vi "main.vi"() -> ()   [LabVIEW 2012]
uses:
  number_of_sources.gbl
  shutter_timeout.gbl
  active_process.gbl
panel:
  in  "Clear elements":bool
  in  "Elements + Rates":cluster{"Elements":u16[], "Rates":sgl[]} {"Rates" min=0 step=0.1 format="%.1f"; "Elements" items=["none", "Ag", "AgBr", "AgCl", "Al", "Al2O3", "Al4C3", "AlF3", "AlN", "AlSb", "As", "As2Se3", "Au", "B", "B2O3", "B4C", "BN", "Ba", "BaF2", "BaN2O6", "BaO", "BaTiO3", "BaTiO3", "Be", "BeF2", "BeO", "Bi", "Bi2O3", "Bi2S3", "Bi2Se3", "Bi2Te3", "BiF3", "C", "C", "C8H8", "Ca", "CaF2", "CaO", "CaO-SiO2", "CaSO4", "CaTiO3", "CaWO4", "Cd", "CdF2", "CdO", "CdS", "CdSe", "CdTe", "Ce", "CeF3", "CeO2", "Co", "CoO", "Cr", "Cr2O3", "Cr3C2", "CrB", "Cs", "Cs2SO4", "CsBr", "CsCl", "CsI", "Cu", "Cu2O", "Cu2S", "Cu2S", "CuS", "Dy", "DY2O3", "Er", "Er2O3", "Eu", "EuF2", "Fe", "Fe2O3", "FeO", "FeS", "Ga", "Ga2O3", "GaAs", "GaN", "GaP", "GaSb", "Gd", "Gd2O3", "Ge", "Ge3N2", "GeO2", "GeTe", "Hf", "HfB2", "HfC", "HfN", "HfO2", "HfSi2", "Hg", "Ho", "Ho2O3", "In", "In2O3", "In2Se3", "In2Te3", "InAs", "InP", "InSb", "Ir", "K", "KBr", "KCl", "KF", "KI", "La", "La2O3", "LaB6", "LaF3", "Li", "LiBr", "LiF", "LiNbO3", "Lu", "Mg", "MgAl2O4", "MgAl2O6", "MgF2", "MgO", "Mn", "MnO", "MnS", "Mo", "Mo2C", "MoB2", "MoO3", "MoS2", "Na", "Na3AlF6", "Na5Al3F14", "NaBr", "NaCl", "NaClO3", "NaF", "NaNO3", "Nb", "Nb2O3", "Nb2O5", "NbB2", "NbC", "NbN", "Nd", "Nd2O3", "NdF3", "Ni", "NiCr", "NiCrFe", "NiFe", "NiFeMo", "NiO", "P3N5", "Pb", "PbCl2", "PbF2", "PbO", "PbS", "PbSe", "PbSnO3", "PbTe", "Pd", "PdO", "Po", "Pr", "Pr2O3", "Pt", "PtO2", "Ra", "Rb", "RbI", "Re", "Rh", "Ru", "S8", "Sb", "Sb2O3", "Sb2S3", "Sc", "Sc2O3", "Se", "Si", "Si3N4", "SiC", "SiO", "SiO2", "Sm", "Sm2O3", "Sn", "SnO2", "SnS", "SnSe", "SnTe", "Sr", "SrF2", "SrO", "Ta", "Ta2O5", "TaB2", "TaC", "TaN", "Tb", "Tc", "Te", "TeO2", "Th", "ThF4", "ThO2", "ThOF2", "Ti", "Ti2O3", "TiB2", "TiC", "TiN", "TiO", "TiO2", "Tl", "TlBr", "TlCl", "TlI", "U", "U3O8", "U4O9", "UO2", "V", "V2O5", "VB2", "VC", "VN", "VO2", "W", "WB2", "WC", "WO3", "WS2", "WSi2", "Y", "Y2O3", "Yb", "Yb2O3", "Zn", "Zn3Sb2", "ZnF2", "ZnO", "ZnS", "ZnSe", "ZnTe", "Zr", "ZrB2", "ZrC", "ZrN", "ZrO2"]}
  in  "Update":bool
  in  "Quit":bool
  in  "Main Menu":cluster{"Deposition":bool, "Deposition 2":bool}
  # "version 1.0.2"
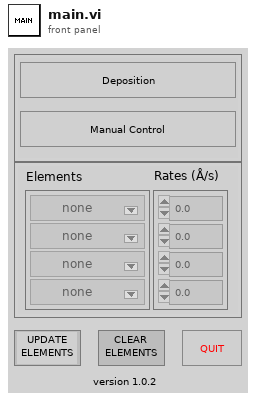
[diagram p1: front panel]
types:
  T1 = cluster{"Active process":i32, "Shutter timeout (ms)":u32, "Number of sources":i32}
  T2 = cluster{"Elements":u16[][], "TD":bool[], "Value":sgl[], "Repeats":i32}[]
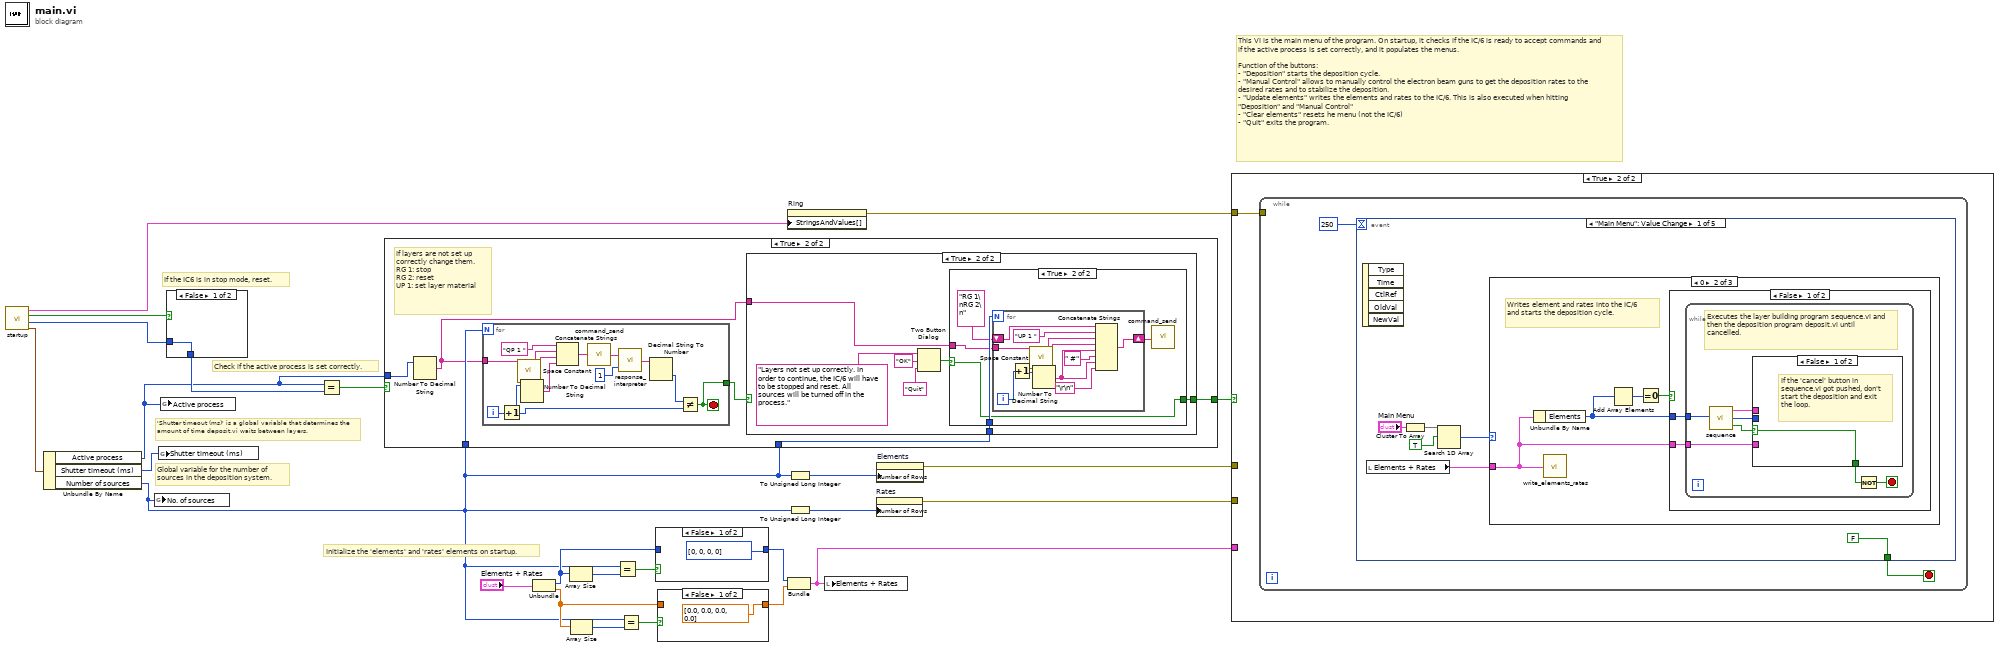
[diagram p0: block diagram]
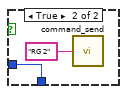
[diagram p2: hidden frame]
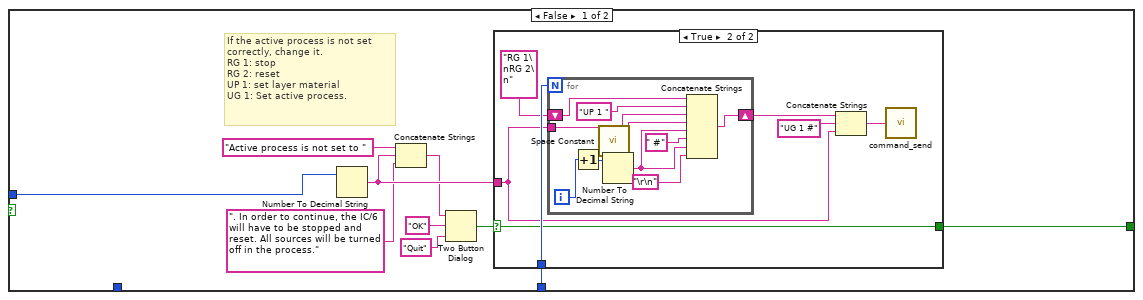
[diagram p3: hidden frame]
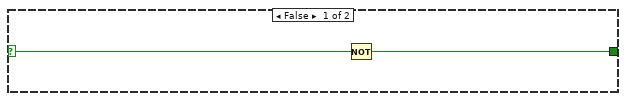
[diagram p5: hidden frame]
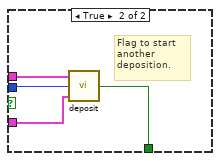
[diagram p9: hidden frame]
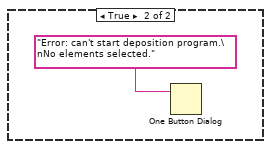
[diagram p10: hidden frame]
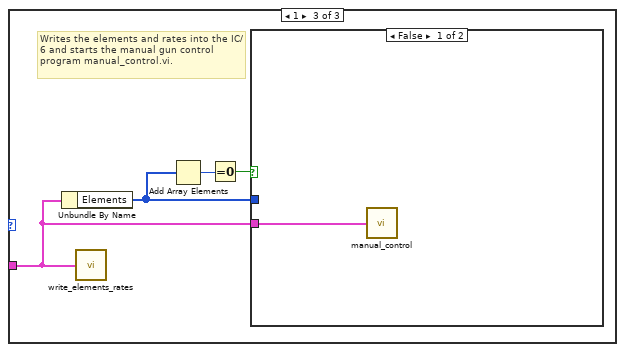
[diagram p11: hidden frame]
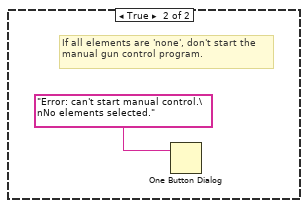
[diagram p12: hidden frame]
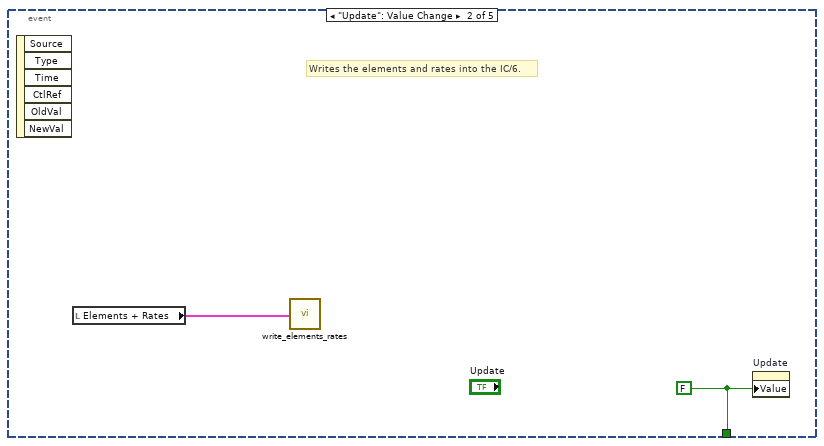
[diagram p13: hidden frame]
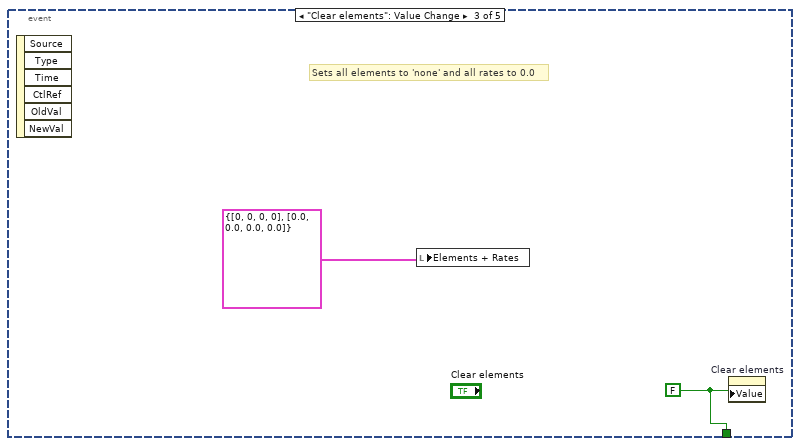
[diagram p14: hidden frame]
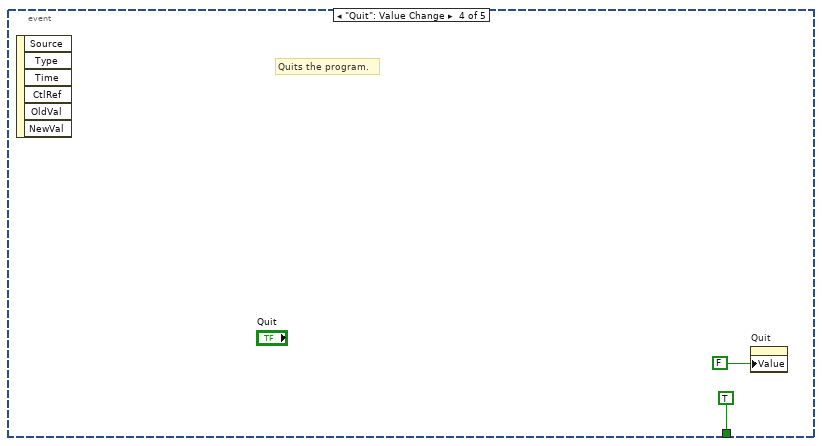
[diagram p15: hidden frame]
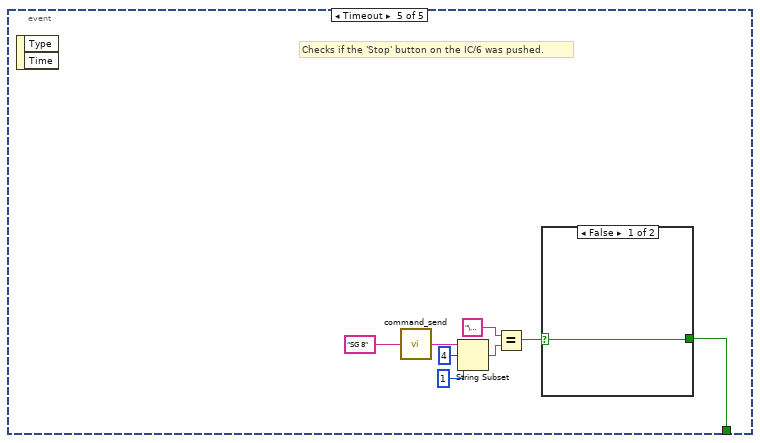
[diagram p16: hidden frame]
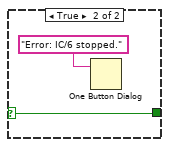
[diagram p17: hidden frame]
diagram:
  # "'Shutter timeout (ms)' is a global variable that determines the amount of time deposit.vi waits between layers."
  # "Global variable for the number of sources in the deposition system."
  # "This VI is the main menu of the program. On startup, it checks if the IC/6 is ready to accept commands and if the active process is set correctly, and it populates the menus.\n\nFunction of the buttons:\n- \"Deposition\" starts the deposition cycle.\n- \"Manual Control\" allows to manually control the electron beam guns to get the deposition rates to the desired rates and to stabilize the deposition.\n- \"Update elements\" writes the elements and rates to the IC/6. This is also executed when hitting \"Deposition\" and \"Manual Control\"\n- \"Clear elements\" resets he menu (not the IC/6)\n- \"Quit\" exits the program."
  # "Check if the active process is set correctly."
  # "If the IC6 is in stop mode, reset."
  # "Initialize the 'elements' and 'rates' elements on startup."
  n1 = call "startup.vi"() -> ("System parameters"=w9:T1, "Active process at IC6"=w10:i32, "Stop?"=w11:bool, "Elements+Rates ring items"=w12:cluster{"Element":string, "Value":u16}[])
  n2 = Unbundle By Name(w9) -> ("Active process"=w5:i32, "Shutter timeout (ms)"=w8:u32, "Number of sources"=w1:i32)
  n3 = global write "number_of_sources.gbl" "No. of sources"(w1) -> ()
  n4 = global write "shutter_timeout.gbl" "Shutter timeout (ms)"(w8) -> ()
  n5 = global write "active_process.gbl" "Active process"(w5) -> ()
  n6 = case shown="False" w11 {
    tunnel: w10 -> [w26 w27]
    tunnel: [w26 w27] -> w7
    frame False {
    }
    frame True {
      n7 = call "command_send.vi"("Commands"="RG 2") -> ()  [unwired: 1 out]
    }
  }
  n8 = Equal?(x=w5, y=w7) -> (x = y?=w20:bool)
  n9 = case shown="True" w20 {
    tunnel: [w35 w61] -> w17
    tunnel: w5 -> [w32 w62]
    tunnel: w1 -> [w29 w60]
    tunnel: w1 -> [_ w58]
    frame False {
      # "If the active process is not set\ncorrectly, change it.\nRG 1: stop\nRG 2: reset\nUP 1: set layer material\nUG 1: Set active process."
      n10 = Number To Decimal String(number=w32) -> (decimal integer string=w33:string)  [unwired: 1 in]
      n11 = Concatenate Strings("Active process is not set to ", w33, ". In order to continue, the IC/6 will have to be stopped and reset. All sources will be turned off in the process.") -> (w30:string)
      n12 = Two Button Dialog(message=w30, 1:"Quit", 2:"OK") -> (T button?=w36:bool)
      n13 = case shown="True" w36 {
        selector: w36 -> [w39 w45]
        tunnel: [w39 w45] -> w35
        tunnel: w33 -> [_ w40]
        tunnel: w29 -> [_ w46]
        frame False {
        }
        frame True {
          n14 = for {
            N: w46 -> [_]
            shift-right: [w56] -> w43
            shift-left: "RG 1\nRG 2\n" -> [w50]
            tunnel: w40 -> [w48]
            i -> [w54]
            n15 = Increment(x=w54) -> (x+1=w55:i32)
            n16 = call <vilib>:"Space Constant.vi"() -> ("String"=w47:string)
            n17 = Number To Decimal String(number=w55) -> (decimal integer string=w52:string)  [unwired: 1 in]
            n18 = Concatenate Strings(w50, "UP 1 ", w48, w47, w52, " #", w52, "\r\n") -> (w56:string)
          }
          n19 = Concatenate Strings(w43, "UG 1 #", w40) -> (w42:string)
          n20 = call "command_send.vi"("Commands"=w42) -> ()  [unwired: 1 out]
        }
      }
    }
    frame True {
      # "If layers are not set up correctly change them.\nRG 1: stop\nRG 2: reset\nUP 1: set layer material"
      n21 = Number To Decimal String(number=w62) -> (decimal integer string=w57:string)  [unwired: 1 in]
      n22 = for {
        N: w58 -> [_]
        tunnel: w57 -> [w70]
        tunnel: [w63] -> w59
        i -> [w74]
        stop <- w63 stop-if-true
        n23 = Increment(x=w74) -> (x+1=w64:i32)
        n24 = call <vilib>:"Space Constant.vi"() -> ("String"=w72:string)
        n25 = Number To Decimal String(number=w64) -> (decimal integer string=w73:string)  [unwired: 1 in]
        n26 = Concatenate Strings("QP 1 ", w70, w72, w73) -> (w67:string)
        n27 = call "command_send.vi"("Commands"=w67) -> ("Response"=w68:string)
        n28 = call "response_interpreter.vi"("Response type"=u16 1, "Response hex"=w68) -> ("Response (readable)"=w66:string)
        n29 = Decimal String To Number(string=w66) -> (number=w65:i32)  [unwired: 2 in, 1 out]
        n30 = Not Equal?(x=w65, y=w64) -> (x != y?=w63:bool)
      }
      n31 = case shown="True" w59 {
        selector: w59 -> [w76 _]
        tunnel: w60 -> [_ w83]
        tunnel: [w75 w82] -> w61
        tunnel: w57 -> [_ w77]
        frame False {
          n32 = Not(x=w76) -> (.not. x?=w75:bool)
        }
        frame True {
          n33 = Two Button Dialog(message="Layers not set up correctly. In order to continue, the IC/6 will have to be stopped and reset. All sources will be turned off in the process.", 1:"Quit", 2:"OK") -> (T button?=w79:bool)
          n34 = case shown="True" w79 {
            selector: w79 -> [w84 w86]
            tunnel: w83 -> [_ w88]
            tunnel: [w84 w86] -> w82
            tunnel: w77 -> [_ w85]
            frame False {
            }
            frame True {
              n35 = for {
                N: w88 -> [_]
                shift-right: [w99] -> w89
                shift-left: "RG 1\nRG 2\n" -> [w93]
                tunnel: w85 -> [w91]
                i -> [w97]
                n36 = Increment(x=w97) -> (x+1=w98:i32)
                n37 = call <vilib>:"Space Constant.vi"() -> ("String"=w90:string)
                n38 = Number To Decimal String(number=w98) -> (decimal integer string=w95:string)  [unwired: 1 in]
                n39 = Concatenate Strings(w93, "UP 1 ", w91, w90, w95, " #", w95, "\r\n") -> (w99:string)
              }
              n40 = call "command_send.vi"("Commands"=w89) -> ()  [unwired: 1 out]
            }
          }
        }
      }
    }
  }
  n41 = Unbundle("Elements + Rates") -> ("Elements"=w3:u16[], "Rates"=w2:sgl[])
  n42 = Array Size(array=w3) -> (size(s)=w18:i32)
  n43 = Array Size(array=w2) -> (size(s)=w19:i32)
  n44 = Equal?(x=w1, y=w18) -> (x = y?=w23:bool)
  n45 = Equal?(x=w1, y=w19) -> (x = y?=w24:bool)
  n46 = case shown="False" w23 {
    tunnel: w3 -> [_ w101]
    tunnel: [u16[] [0, 0, 0, 0] w101] -> w21
    frame False {
    }
    frame True {
    }
  }
  n47 = case shown="False" w24 {
    tunnel: w2 -> [_ w103]
    tunnel: [sgl[] [0.0, 0.0, 0.0, 0.0] w103] -> w22
    frame False {
    }
    frame True {
    }
  }
  n48 = property on="Ring" class="Ring (strict)"("StringsAndValues[]"=w12) -> (error out=w16:errorcluster)  [unwired: 2 in, 1 out]
  n49 = Bundle("Elements"=w21, "Rates"=w22) -> (w13:cluster{"Elements":u16[], "Rates":sgl[]})  [unwired: 1 in]
  n50 = To Unsigned Long Integer(number=w1) -> (unsigned 32bit integer=w4:u32)
  n51 = To Unsigned Long Integer(number=w1) -> (unsigned 32bit integer=w6:u32)
  n52 = local write "Elements + Rates"(w13) -> ()
  n53 = property on="Rates" class="Arr (strict)"("Number of Rows"=w6) -> (error out=w14:errorcluster)  [unwired: 2 in, 1 out]
  n54 = property on="Elements" class="Arr (strict)"("Number of Rows"=w4) -> (error out=w15:errorcluster)  [unwired: 2 in, 1 out]
  n55 = case shown="True" w17 {
    tunnel: w16 -> [_ w104]
    tunnel: w15 -> [_ _]
    tunnel: w14 -> [_ _]
    tunnel: w13 -> [_ _]
    frame False {
    }
    frame True {
      n56 = while {
        tunnel: w104 -> [_]
        stop <- w106 stop-if-true
        n57 = event shown="[0] \"Main Menu\": Value Change" {
          selector: _ -> [_ _ _ _ _]
          dyn-events: _ -> [_ _ _ _ _]
          timeout: 250 -> [_ _ _ _ _]
          tunnel: [FALSE w138 w140 TRUE w145] -> w106
          event "Main Menu": Value Change {
            n58 = event-data() -> ()  [unwired: 1 in, 5 out]
            n59 = local read "Elements + Rates"() -> (w107:cluster{"Elements":u16[], "Rates":sgl[]})
            n60 = Cluster To Array(cluster="Main Menu") -> (array=w111:bool[])
            n61 = Search 1D Array(1D array=w111, element=TRUE) -> (index of element=w109:i32)  [unwired: 1 in]
            n62 = case shown="0" w109 {
              tunnel: w107 -> [_ w113 w132]
              frame -1, Default {
              }
              frame 0 {
                # "Writes element and rates into the IC/6 and starts the deposition cycle."
                n63 = Unbundle By Name(w113) -> ("Elements"=w114:u16[])
                n64 = call "write_elements_rates.vi"("Elements + Rates"=w113) -> ()
                n65 = Add Array Elements(numeric array=w114) -> (sum=w115:u16)
                n66 = Equal To 0?(x=w115) -> (x = 0?=w116:bool)
                n67 = case shown="False" w116 {
                  tunnel: w114 -> [w118 _]
                  tunnel: w113 -> [w117 _]
                  frame False {
                    n68 = while {
                      tunnel: w118 -> [w120]
                      tunnel: w117 -> [w119]
                      stop <- w124 stop-if-true
                      # "Executes the layer building program sequence.vi and then the deposition program deposit.vi until cancelled."
                      n69 = call "sequence.vi"("Elements@IC6"=w120) -> ("Output Array"=w123:T2, "# of layers"=w121:i32, "Start/Cancel"=w122:bool)
                      n70 = case shown="False" w122 {
                        selector: w122 -> [w126 _]
                        tunnel: [w126 w129] -> w125
                        tunnel: w123 -> [_ w130]
                        tunnel: w121 -> [_ w128]
                        tunnel: w119 -> [_ w127]
                        frame False {
                          # "If the 'cancel' button in sequence.vi got pushed, don't start the deposition and exit the loop."
                        }
                        frame True {
                          # "Flag to start another deposition."
                          n71 = call "deposit.vi"("Elements+Rates"=w127, "# of units"=w128, "Input array"=w130) -> ("Deposit again?"=w129:bool)
                        }
                      }
                      n72 = Not(x=w125) -> (.not. x?=w124:bool)
                    }
                  }
                  frame True {
                    n73 = One Button Dialog(message="Error: can't start deposition program.\nNo elements selected.") -> ()  [unwired: 1 in, 1 out]
                  }
                }
              }
              frame 1 {
                # "Writes the elements and rates into the IC/6 and starts the manual gun control program manual_control.vi."
                n74 = Unbundle By Name(w132) -> ("Elements"=w133:u16[])
                n75 = call "write_elements_rates.vi"("Elements + Rates"=w132) -> ()
                n76 = Add Array Elements(numeric array=w133) -> (sum=w135:u16)
                n77 = Equal To 0?(x=w135) -> (x = 0?=w134:bool)
                n78 = case shown="False" w134 {
                  tunnel: w133 -> [_ _]
                  tunnel: w132 -> [w136 _]
                  frame False {
                    n79 = call "manual_control.vi"("Elements+Rates"=w136) -> ()
                  }
                  frame True {
                    # "If all elements are 'none', don't start the manual gun control program."
                    n80 = One Button Dialog(message="Error: can't start manual control.\nNo elements selected.") -> ()  [unwired: 1 in, 1 out]
                  }
                }
              }
            }
          }
          event "Update": Value Change {
            w138 = FALSE
            # "Writes the elements and rates into the IC/6."
            n81 = event-data() -> ()  [unwired: 1 in, 6 out]
            n82 = local read "Elements + Rates"() -> (w139:cluster{"Elements":u16[], "Rates":sgl[]})
            n83 = call "write_elements_rates.vi"("Elements + Rates"=w139) -> ()
            n84 = property on="Update" class="Bool (strict)"("Value"=w138) -> ()  [unwired: 2 in, 2 out]
          }
          event "Clear elements": Value Change {
            w140 = FALSE
            # "Sets all elements to 'none' and all rates to 0.0"
            n85 = event-data() -> ()  [unwired: 1 in, 6 out]
            n86 = local write "Elements + Rates"(cluster{u16[], sgl[]} {[0, 0, 0, 0], [0.0, 0.0, 0.0, 0.0]}) -> ()
            n87 = property on="Clear elements" class="Bool (strict)"("Value"=w140) -> ()  [unwired: 2 in, 2 out]
          }
          event "Quit": Value Change {
            # "Quits the program."
            n88 = event-data() -> ()  [unwired: 1 in, 6 out]
            n89 = property on="Quit" class="Bool (strict)"("Value"=FALSE) -> ()  [unwired: 2 in, 2 out]
          }
          event Timeout {
            # "Checks if the 'Stop' button on the IC/6 was pushed."
            n90 = event-data() -> ()  [unwired: 1 in, 2 out]
            n91 = call "command_send.vi"("Commands"="SG 8") -> ("Response"=w150:string)
            n92 = String Subset(string=w150, offset (0)=4, length (rest)=1) -> (substring=w147:string)
            n93 = Equal?(x="\u0006", y=w147) -> (x = y?=w146:bool)
            n94 = case shown="False" w146 {
              selector: w146 -> [w152 w153]
              tunnel: [w152 w153] -> w145
              frame False {
              }
              frame True {
                n95 = One Button Dialog(message="Error: IC/6 stopped.") -> ()  [unwired: 1 in, 1 out]
              }
            }
          }
        }
      }
    }
  }
